vi "convert_unit_set.vi"(8 "error in (no error)":errorcluster, 11 "raw_data []":T2(array[cluster])) -> (0 "error out":errorcluster, 3 "units []":T1[](array[typedef]))   [LabVIEW 2015, in "lv-unit-conversion.lvlib"]
uses:
  lv-unit-conversion.lvlib
  _controls/unit_set.ctl
  _controls/error.ctl
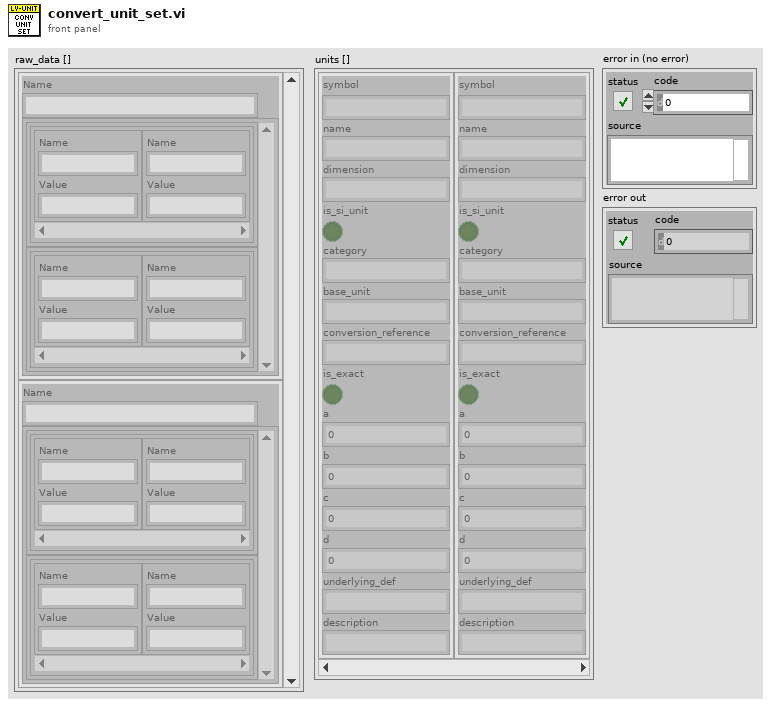
[diagram p1: front panel]
types:
  T1 = typedef "lv-unit-conversion.lvlib/unit_set.ctl" = cluster{"symbol":string, "name":string, "dimension":string, "is_si_unit":bool, "category":string, "base_unit":string, "conversion_reference":string, "is_exact":bool, "a":dbl, "b":dbl, "c":dbl, "d":dbl, "underlying_def":string, "description":string}
  T2 = cluster{"Name":string, cluster{cluster{"Name":string, "Value":string}[]}[]}[]
  T3 = typedef "lv-unit-conversion.lvlib/error.ctl" = enum16{"<lv-unit-conversion_error>", "unit_not_found", "xml_parser", "set_not_found", "<null>"}
  T4 = cluster{cluster{"Name":string, "Value":string}[]}[]
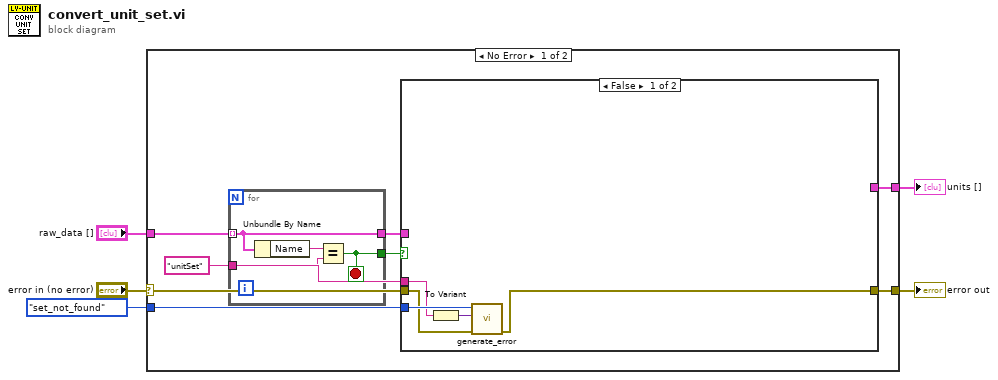
[diagram p0: block diagram]
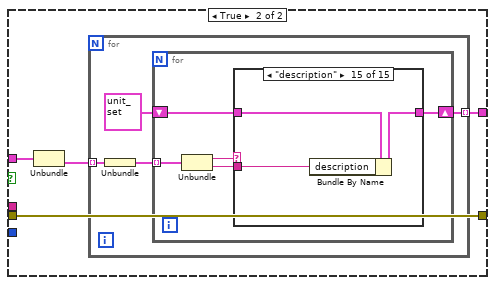
[diagram p2: hidden frame]
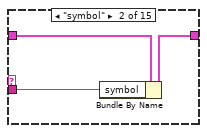
[diagram p4: hidden frame]
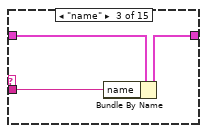
[diagram p5: hidden frame]
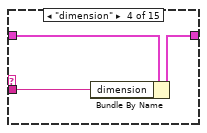
[diagram p6: hidden frame]
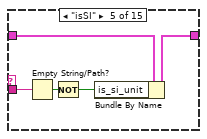
[diagram p7: hidden frame]
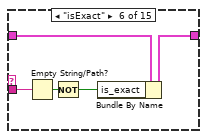
[diagram p8: hidden frame]
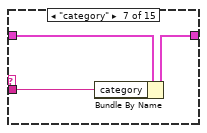
[diagram p9: hidden frame]
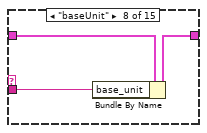
[diagram p10: hidden frame]
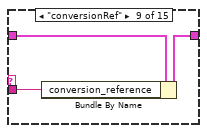
[diagram p11: hidden frame]
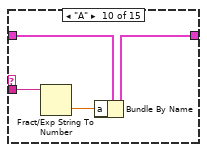
[diagram p12: hidden frame]
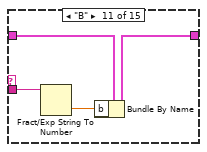
[diagram p13: hidden frame]
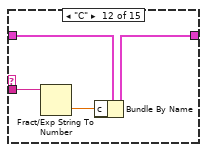
[diagram p14: hidden frame]
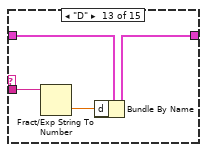
[diagram p15: hidden frame]
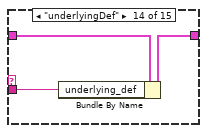
[diagram p16: hidden frame]
diagram:
  n1 = case shown="No Error" "error in (no error)" {
    selector: "error in (no error)" -> [w9 w87]
    tunnel: "raw_data []" -> [w12 _]
    tunnel: [w11 _] -> w4
    tunnel: [w8 w87] -> w2
    tunnel: error."set_not_found" ("error") -> [w7 _]
    frame No Error {
      w6 = "unitSet" ("Name")
      n2 = for {
        tunnel: w12 -> [w17] mode=indexing
        tunnel: [w17] -> w10
        tunnel: [w15] -> w13
        tunnel: w6 -> [w14]
        stop <- w15 stop-if-true
        n3 = Unbundle By Name(w17) -> ("Name"=w16:string)
        n4 = Equal?(x=w16, y=w14) -> (x = y?=w15:bool)
      }
      n5 = case shown="False" w13 {
        tunnel: w10 -> [_ w26]
        tunnel: [_ w24] -> w11
        tunnel: w9 -> [w21 w23]
        tunnel: [w20 w23] -> w8
        tunnel: w7 -> [w22 _]
        tunnel: w6 -> [w19 _]
        frame False {
          n6 = To Variant(anything=w19) -> (Variant=w18:variant)
          n7 = call "generate_error.vi"("error in (no error)"=w21, "data"=w18, "error"=w22) -> ("error out"=w20:errorcluster)  [unwired: 8 in]
        }
        frame True {
          n8 = Unbundle(w26) -> (w25:T4)  [unwired: 1 out]
          n9 = for {
            tunnel: w25 -> [w30] mode=indexing
            tunnel: [w27] -> w24 mode=indexing
            n10 = Unbundle(w30) -> (w29:cluster{"Name":string, "Value":string}[])
            n11 = for {
              tunnel: w29 -> [w35] mode=indexing
              shift-right: [w31] -> w27
              shift-left: T1 {"symbol"="", "name"="", "dimension"="", "is_si_unit"=FALSE, "category"="", "base_unit"="", "conversion_reference"="", "is_exact"=FALSE, "a"=0.0, "b"=0.0, "c"=0.0, "d"=0.0, "underlying_def"="", "description"=""} ("unit_set") -> [w32]
              n12 = Unbundle(w35) -> ("Name"=w34:string, "Value"=w33:string)
              n13 = case shown="\"description\"" w34 {
                tunnel: w33 -> [_ w37 w40 w43 w48 w53 w56 w59 w62 w66 w70 w74 w78 w81 w84]
                tunnel: w32 -> [w36 w39 w42 w45 w50 w55 w58 w61 w64 w68 w72 w76 w80 w83 w86]
                tunnel: [w36 w38 w41 w44 w49 w54 w57 w60 w63 w67 w71 w75 w79 w82 w85] -> w31
                frame Default {
                }
                frame "symbol" {
                  n14 = Bundle By Name(cluster=w39, "symbol"=w37) -> (w38:T1)
                }
                frame "name" {
                  n15 = Bundle By Name(cluster=w42, "name"=w40) -> (w41:T1)
                }
                frame "dimension" {
                  n16 = Bundle By Name(cluster=w45, "dimension"=w43) -> (w44:T1)
                }
                frame "isSI" {
                  n17 = Empty String/Path?(string/path=w48) -> (empty?=w47:bool)
                  n18 = Not(x=w47) -> (.not. x?=w46:bool)
                  n19 = Bundle By Name(cluster=w50, "is_si_unit"=w46) -> (w49:T1)
                }
                frame "isExact" {
                  n20 = Empty String/Path?(string/path=w53) -> (empty?=w52:bool)
                  n21 = Not(x=w52) -> (.not. x?=w51:bool)
                  n22 = Bundle By Name(cluster=w55, "is_exact"=w51) -> (w54:T1)
                }
                frame "category" {
                  n23 = Bundle By Name(cluster=w58, "category"=w56) -> (w57:T1)
                }
                frame "baseUnit" {
                  n24 = Bundle By Name(cluster=w61, "base_unit"=w59) -> (w60:T1)
                }
                frame "conversionRef" {
                  n25 = Bundle By Name(cluster=w64, "conversion_reference"=w62) -> (w63:T1)
                }
                frame "A" {
                  n26 = Fract/Exp String To Number(string=w66) -> (number=w65:dbl)  [unwired: 3 in, 1 out]
                  n27 = Bundle By Name(cluster=w68, "a"=w65) -> (w67:T1)
                }
                frame "B" {
                  n28 = Fract/Exp String To Number(string=w70) -> (number=w69:dbl)  [unwired: 3 in, 1 out]
                  n29 = Bundle By Name(cluster=w72, "b"=w69) -> (w71:T1)
                }
                frame "C" {
                  n30 = Fract/Exp String To Number(string=w74) -> (number=w73:dbl)  [unwired: 3 in, 1 out]
                  n31 = Bundle By Name(cluster=w76, "c"=w73) -> (w75:T1)
                }
                frame "D" {
                  n32 = Fract/Exp String To Number(string=w78) -> (number=w77:dbl)  [unwired: 3 in, 1 out]
                  n33 = Bundle By Name(cluster=w80, "d"=w77) -> (w79:T1)
                }
                frame "underlyingDef" {
                  n34 = Bundle By Name(cluster=w83, "underlying_def"=w81) -> (w82:T1)
                }
                frame "description" {
                  n35 = Bundle By Name(cluster=w86, "description"=w84) -> (w85:T1)
                }
              }
            }
          }
        }
      }
    }
    frame Error {
    }
  }
  "units []" <- w4
  "error out" <- w2
